vi "Generate Event to View Core.vi"(9 "Event in":refnum<class "Event.lvclass">, 10 "Event Handler Details":T1, 11 "Message Enqueuer in":refnum<class "Message Enqueuer.lvclass">) -> ()   [LabVIEW 2023, in "Event Actors.lvlib" / "Controller Actor.lvclass"]
uses:
  Controller Actor.lvclass
  <vilib>/ActorFramework/Message Enqueuer/Message Enqueuer.lvclass
  Event/Event.lvclass
  Event Handler Details.ctl
  Event Handlers/Abstract Event Message for View/Abstract Event Message for View.lvclass
  C:/Program Files/National Instruments/LabVIEW 2023/vi.lib/ActorFramework/Message/Message.lvclass
  Event Handlers/Abstract Event Message for View/Abstract Event Message for View.lvclass/Abstract Event Message for View.ctl
  <vilib>/ActorFramework/Message Enqueuer/Message Enqueuer.lvclass/Message Enqueuer.ctl
  <vilib>/ActorFramework/Message Enqueuer/Enqueue.vi
  <vilib>/Utility/LVClass/Get LV Class Name.vi
  <resource>/AFDebug/Generate Trace for Message.vi
  <vilib>/ActorFramework/Message Priority Queue/Priority Enqueue.vi
  Controller Actor.lvclass/Controller Actor.ctl
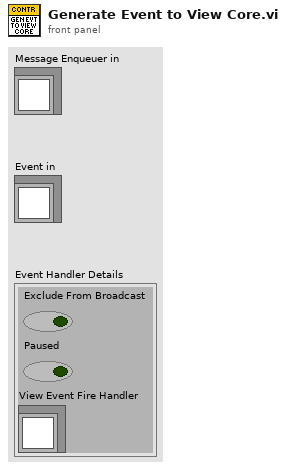
[diagram p1: front panel]
types:
  T1 = typedef "Event Actors.lvlib/Controller Actor.lvclass/Event Handler Details.ctl" = cluster{"Exclude From Broadcast":bool, "Paused":bool, "View Event Fire Handler":refnum<class "Abstract Event Message for View.lvclass">}
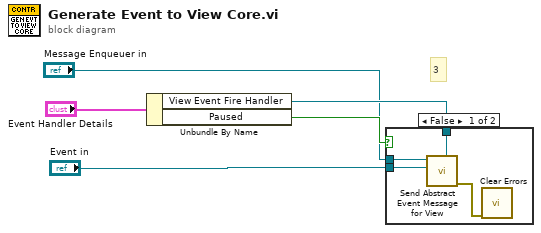
[diagram p0: block diagram]
diagram:
  # "3"
  n1 = Unbundle By Name("Event Handler Details") -> ("View Event Fire Handler"=w4:refnum<class "Abstract Event Message for View.lvclass">, "Paused"=w5:bool)
  n2 = case shown="False" w5 {
    tunnel: w4 -> [w9 _]
    tunnel: "Event in" -> [w8 _]
    tunnel: "Message Enqueuer in" -> [w6 _]
    frame False {
      n3 = call "Send Abstract Event Message for View.vi"("Message Type"=w9, "Event Data"=w8, "Message Enqueuer"=w6) -> ("Error Out"=w7:errorcluster)  [unwired: 7 in, 1 out]
      n4 = call <vilib>:"Clear Errors.vi"("error in (no error)"=w7) -> ()  [unwired: 5 in, 2 out]
    }
    frame True {
    }
  }
